vi "DIAdem Script Command.vi"(6 "Script Path (\"\")":path, 8 "error in (no error)":errorcluster, 9 "Parameter (\"\")":string, 10 "Command (\"\")":string, 11 "DIAdem Reference":T1) -> (0 "error out":errorcluster, 3 "dup DIAdem Reference":T1)   [LabVIEW 2011]
uses:
  <vilib>/addons/DIAdem/DIAdem.llb/DIAdem Reference.ctl
  <vilib>/addons/DIAdem/DIAdem.llb/DIAdem String Variable Set.vi
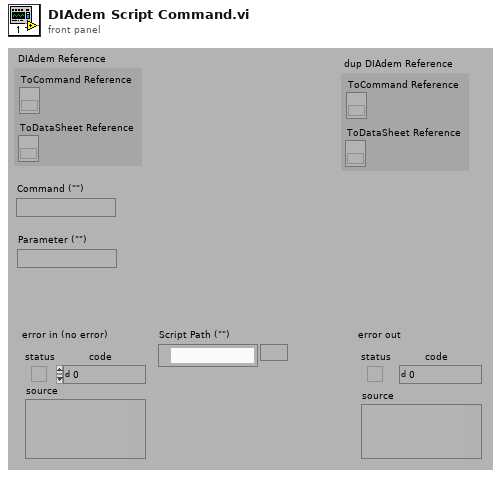
[diagram p1: front panel]
types:
  T1 = typedef "DIAdem Reference.ctl" = cluster{"ToCommand Reference":refnum<k7>, "ToDataSheet Reference":refnum<k7>}
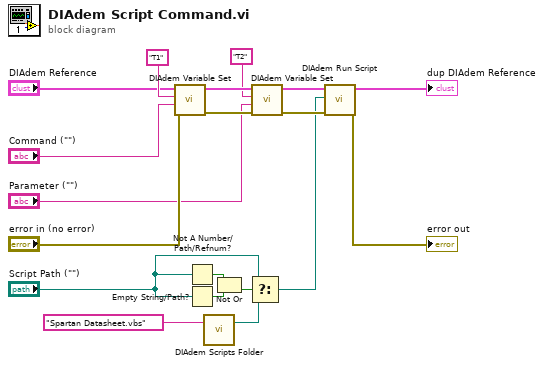
[diagram p0: block diagram]
diagram:
  n1 = call-poly <vilib>:"DIAdem Variable Set.vi"("error in (no error)"="error in (no error)", "Value"="Command (\"\")", "Variable Name"="T1", "DIAdem Reference"="DIAdem Reference") -> ("error out"=w16:errorcluster, "DIAdem Reference"=w18:T1)  [unwired: 6 out]
  n2 = Not A Number/Path/Refnum?(number/path/refnum="Script Path (\"\")") -> (NaN/Path/Refnum?=w3:bool)
  n3 = Empty String/Path?(string/path="Script Path (\"\")") -> (empty?=w4:bool)
  n4 = call "DIAdem Scripts Folder.vi"("Relative Path (\"\" - Folder)"="Spartan Datasheet.vbs" ("Object Name (\"\")")) -> ("Scripts Folder"=w5:path)  [unwired: 2 out]
  n5 = Not Or(1:w4, 2:w3) -> (0:w2:bool)
  n6 = Select(t="Script Path (\"\")", s=w2, f=w5) -> (s? t:f=w9:path)
  n7 = call-poly <vilib>:"DIAdem Variable Set.vi"("error in (no error)"=w16, "Value"="Parameter (\"\")", "Variable Name"="T2", "DIAdem Reference"=w18) -> ("error out"=w15:errorcluster, "DIAdem Reference"=w17:T1)  [unwired: 6 out]
  n8 = call <vilib>:"DIAdem Run Script.vi"("error in (no error)"=w15, "script file"=w9, "DIAdem Reference"=w17) -> ("error out"=→"error out":errorcluster, "DIAdem Reference"=→"dup DIAdem Reference":T1)  [unwired: 7 out]
